vi "Destroy.vi"(8 "error in":errorcluster, 11 "BufferLossless in":refnum<class "BufferLossless.lvclass">) -> (0 "error out":errorcluster, 3 "BufferLossless out":refnum<class "BufferLossless.lvclass">)   [LabVIEW 2024, in "BufferLossless.lvclass"]
uses:
  BufferLossless.lvclass
  BufferLossless.lvclass/BufferLossless.ctl
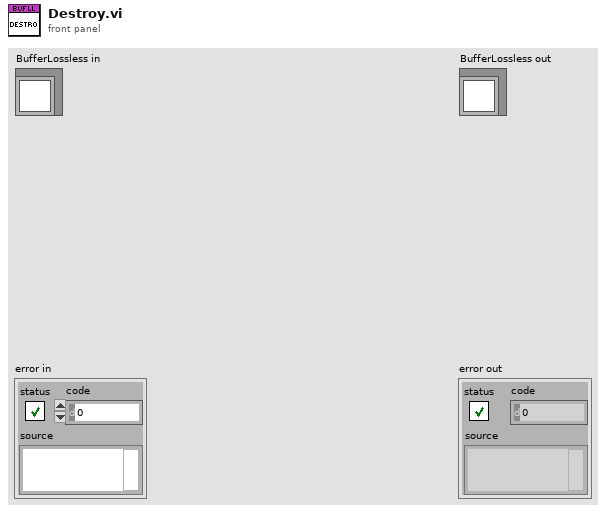
[diagram p1: front panel]
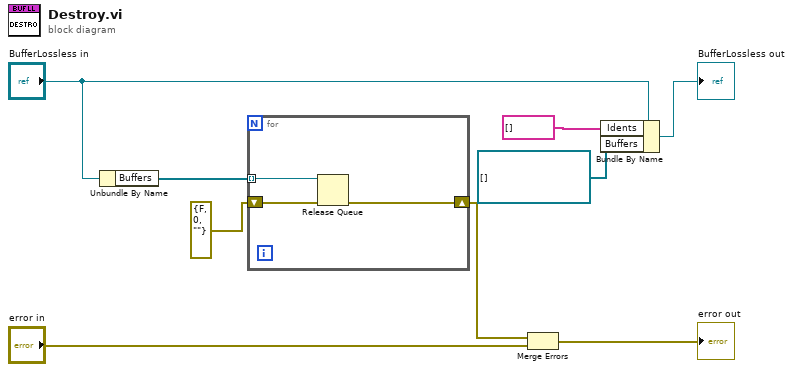
[diagram p0: block diagram]
diagram:
  n1 = Unbundle By Name("BufferLossless in") -> ("Buffers"=w8:refnum<queue>[])
  n2 = for {
    tunnel: w8 -> [w12] mode=indexing
    shift-right: [w11] -> w5
    shift-left: errorcluster {"status"=FALSE, "code"=0, "source"=""} ("error out") -> [w10]
    n3 = Release Queue(queue=w12, error in (no error)=w10) -> (error out=w11:errorcluster)  [unwired: 1 in, 2 out]
  }
  n4 = Merge Errors(w5, "error in") -> (→"error out":errorcluster)
  n5 = Bundle By Name(cluster="BufferLossless in", "Idents"=string[] [], "Buffers"=refnum<queue>[] []) -> (→"BufferLossless out":refnum<class "BufferLossless.lvclass">)
